vi "Accel_Test.vi"() -> ()   [LabVIEW 2015]
uses:
  <vilib>/myRIO/Instrument Drivers/Onboard Devices/Accelerometer/typedefs/Accelerometer Reference.ctl
  <vilib>/myRIO/Common/Instrument Driver Framework/Utilities/typedefs/myRIO Generic Hardware Reference.ctl
  <vilib>/myRIO/Common/Instrument Driver Framework/Utilities/typedefs/Hardware Version Enum.ctl
  <vilib>/myRIO/Common/Instrument Driver Framework/Utilities/typedefs/myRIO v1.0 Reference.ctl
  <vilib>/myRIO/Common/Instrument Driver Framework/Utilities/typedefs/Generic FPGA Reference.ctl
  <vilib>/myRIO/Common/Instrument Driver Framework/myRIO v1.0/Accelerometer/typedefs/Accelerometer Channels List.ctl
  <vilib>/myRIO/Common/Instrument Driver Framework/myRIO v1.0/Accelerometer/typedefs/Accelerometer Channels Enum.ctl
  <vilib>/userdefined/High Color/nirio_resource_hc.ctl
  <vilib>/myRIO/Common/Instrument Driver Framework/Utilities/vis/Is FPGA Ref Available.vi
  <vilib>/myRIO/Common/Instrument Driver Framework/myRIO v1.0/Accelerometer/vis/myRIO v1.1 Open Accelerometer.vi
  <vilib>/myRIO/Instrument Drivers/Onboard Devices/Accelerometer/vis/Read.vi
  <vilib>/Analysis/8numeric.llb/1D Numeric Integration.vi
  <vilib>/myRIO/Common/Instrument Driver Framework/Utilities/vis/Validate Channels.vi
  <vilib>/myRIO/Common/Instrument Driver Framework/myRIO v1.0/Accelerometer/vis/myRIO v1.0 Reserve Accelerometer.vi
  <vilib>/myRIO/Common/Instrument Driver Framework/myRIO v1.0/Resource Manager/vis/myRIO v1.0 Reserve Channel List.vi
  <vilib>/myRIO/Common/Instrument Driver Framework/myRIO v1.0/Accelerometer/vis/myRIO v1.0 Build MUX Configuration Accelerometer.vi
  <vilib>/myRIO/Common/Instrument Driver Framework/myRIO v1.0/Resource Manager/vis/myRIO v1.0 Reserve Channel.vi
  <vilib>/myRIO/Common/Instrument Driver Framework/myRIO v1.0/Resource Manager/vis/myRIO v1.0 Unreserve Channel.vi
  <vilib>/myRIO/Common/Instrument Driver Framework/myRIO v1.0/Resource Manager/vis/myRIO v1.0 Build Mutex Name.vi
  <vilib>/Utility/VariantDataType/GetNumericInfo.vi
  <vilib>/Utility/error.llb/Error Cluster From Error Code.vi
  <vilib>/myRIO/Common/Instrument Driver Framework/myRIO v1.0/myRIO v1.1 Open.vi
  <vilib>/myRIO/Common/Instrument Driver Framework/myRIO v1.0/Accelerometer/vis/myRIO v1.0 Get Scaling Constant Accelerometer.vi
  <vilib>/myRIO/Common/Instrument Driver Framework/Utilities/vis/IO Manager.vi
  <vilib>/myRIO/Common/Instrument Driver Framework/Utilities/vis/Configuration Manager.vi
  <vilib>/myRIO/Common/Instrument Driver Framework/myRIO v1.0/myRIO v1.0 Close.vi
  <vilib>/myRIO/Common/Instrument Driver Framework/myRIO v1.0/Accelerometer/vis/myRIO v1.0 Read Accelerometer.vi
  <vilib>/myRIO/Express VI/Onboard Devices/Accelerometer/Accelerometer Express VI.xnode
  <vilib>/myRIO/Instrument Drivers/Onboard Devices/Accelerometer/vis/myRIO Accelerometer Open.xnode
  <vilib>/Analysis/NI_AALPro.lvlib
  <vilib>/myRIO/Instrument Drivers/Onboard Devices/Accelerometer/Accelerometer.lvlib
panel:
  out "Waveform Chart  Y  2":dbl(graph)
  out "X-Axis 3":dbl
  out "dX/dY  Chart 3":dbl(graph)
  out "x/y":dbl
  out "Waveform Chart  Y":dbl(graph)
  out "Y-Axis":dbl
  out "\"position\"":dbl(graph)
  out "Current V":dbl
  out "Current A":dbl
  out "dX":dbl(graph)
  out "dA":dbl(graph)
  out "Avg A":dbl(graph)
  in  "stop 2":bool
  out "X-Axis 2":dbl
  out "Waveform Chart 2":dbl(graph)
  out "Waveform Chart X":dbl(graph)
  out "X-Axis":dbl
  in  "stop":bool
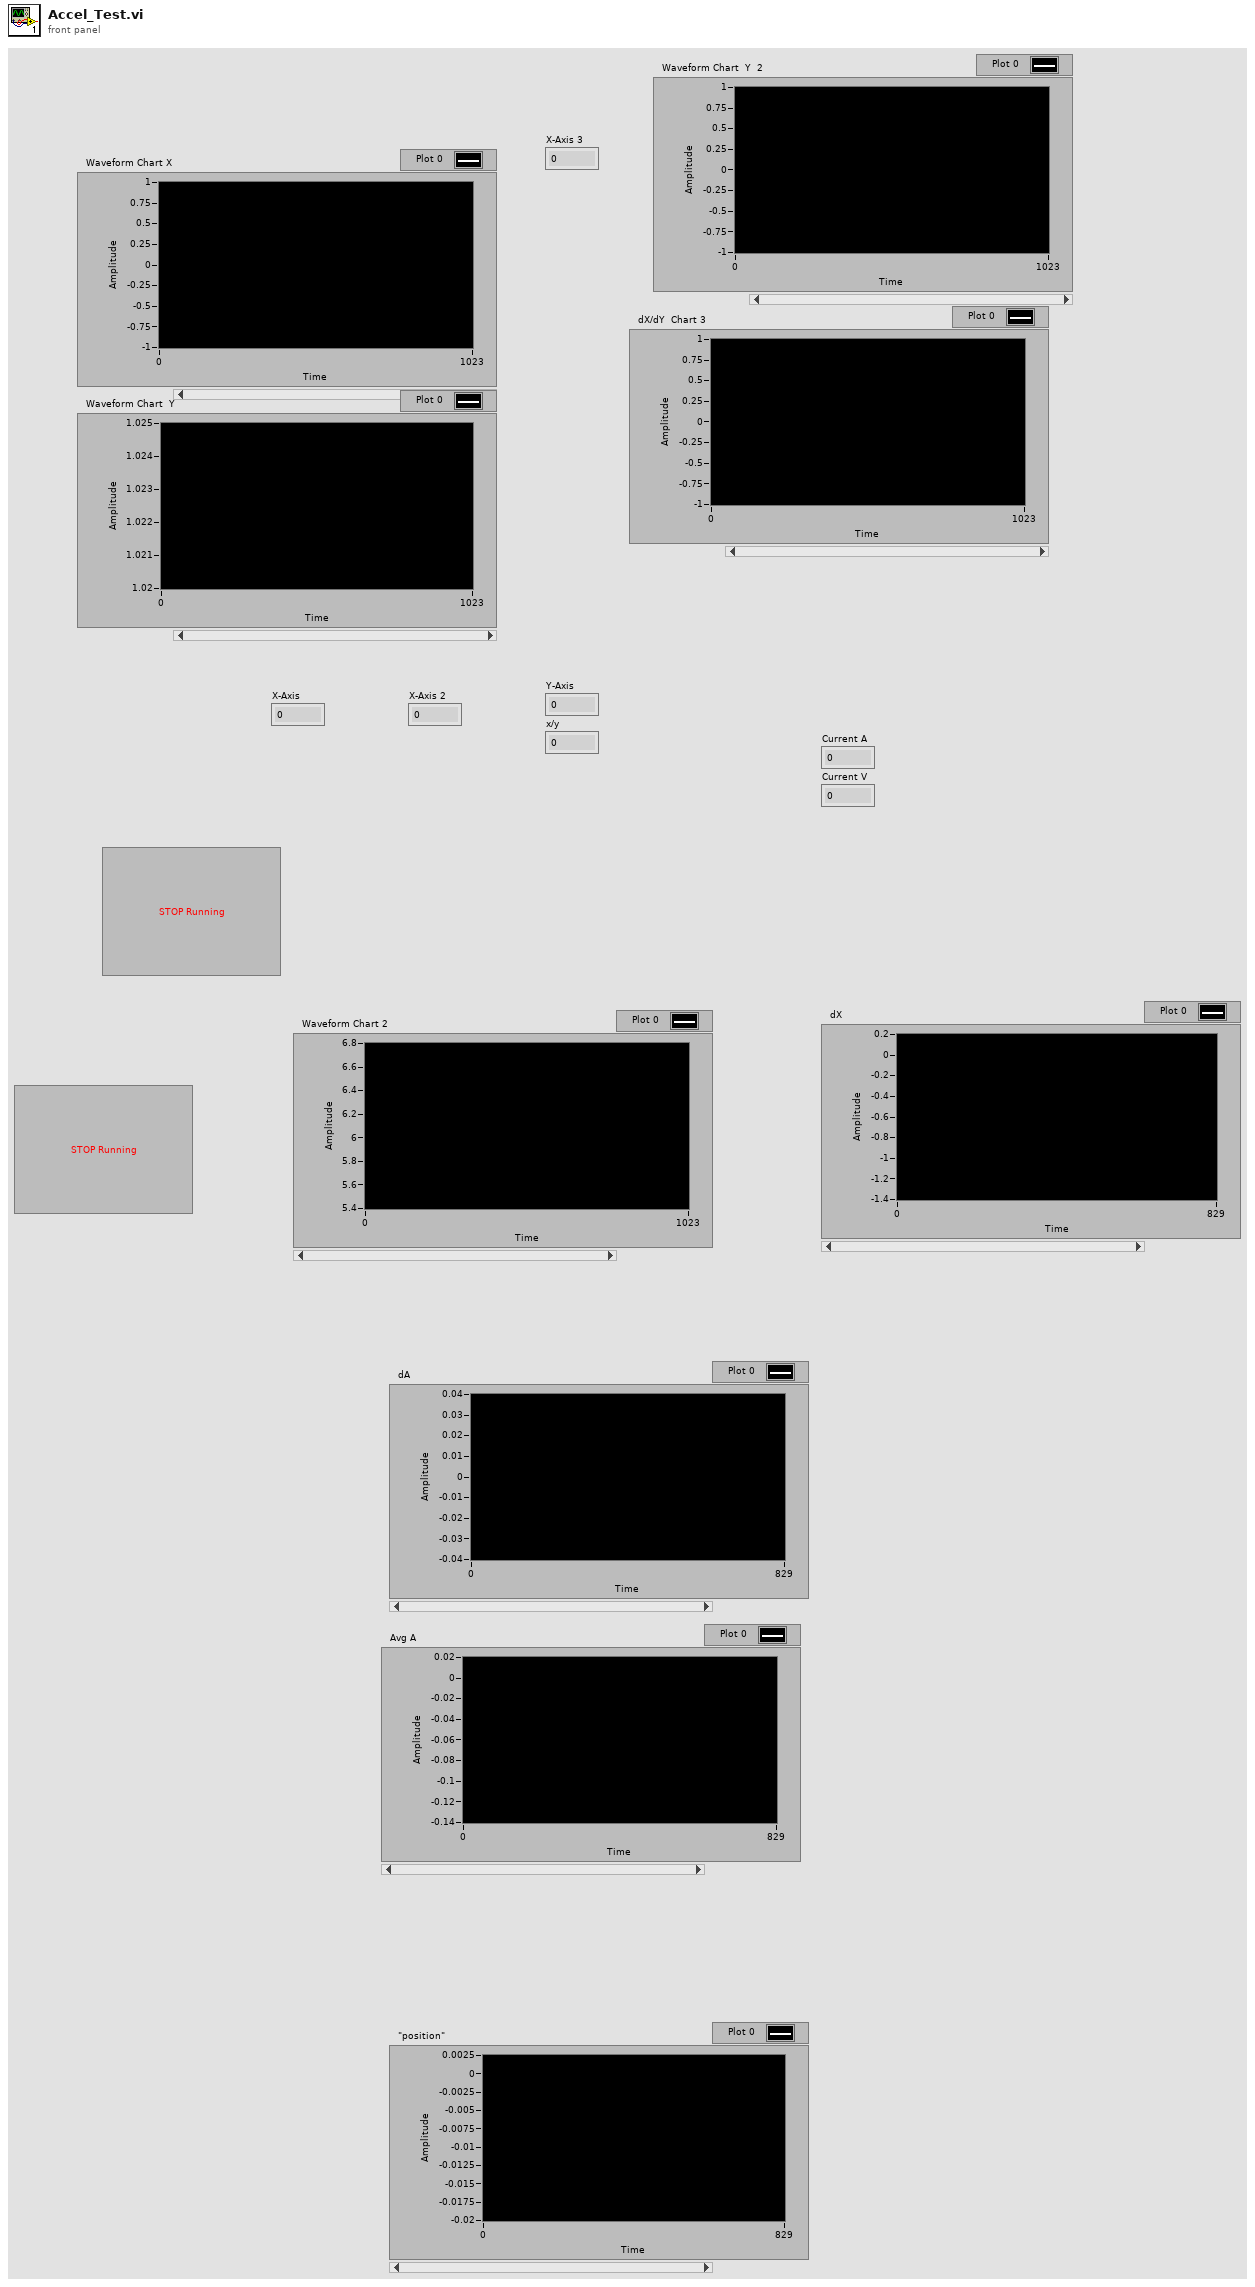
[diagram p1: front panel]
types:
  T1 = typedef "Accelerometer.lvlib/Accelerometer Reference.ctl" = cluster{"myRIO Reference":T2, "Accelerometer Channels List":T6, "LSB Weight":dbl}
  T2 = typedef "myRIO Generic Hardware Reference.ctl" = cluster{"myRIO Model":T3, "myRIO Hardware Reference":T4}
  T3 = typedef "Hardware Version Enum.ctl" = enum16{"Unknown", "myRIO-1900", "myRIO-1950", "roboRIO"}
  T4 = typedef "myRIO v1.0 Reference.ctl" = cluster{"Generic FPGA Reference":T5, "Allow multiple opens":bool}
  T5 = typedef "Generic FPGA Reference.ctl" = refnum<k20>
  T6 = typedef "Accelerometer Channels List.ctl" = T7[]
  T7 = typedef "Accelerometer Channels Enum.ctl" = enum16{"Not Connected", "X-Axis", "Y-Axis", "Z-Axis"}
  T8 = typedef "nirio_resource_hc.ctl" = tag
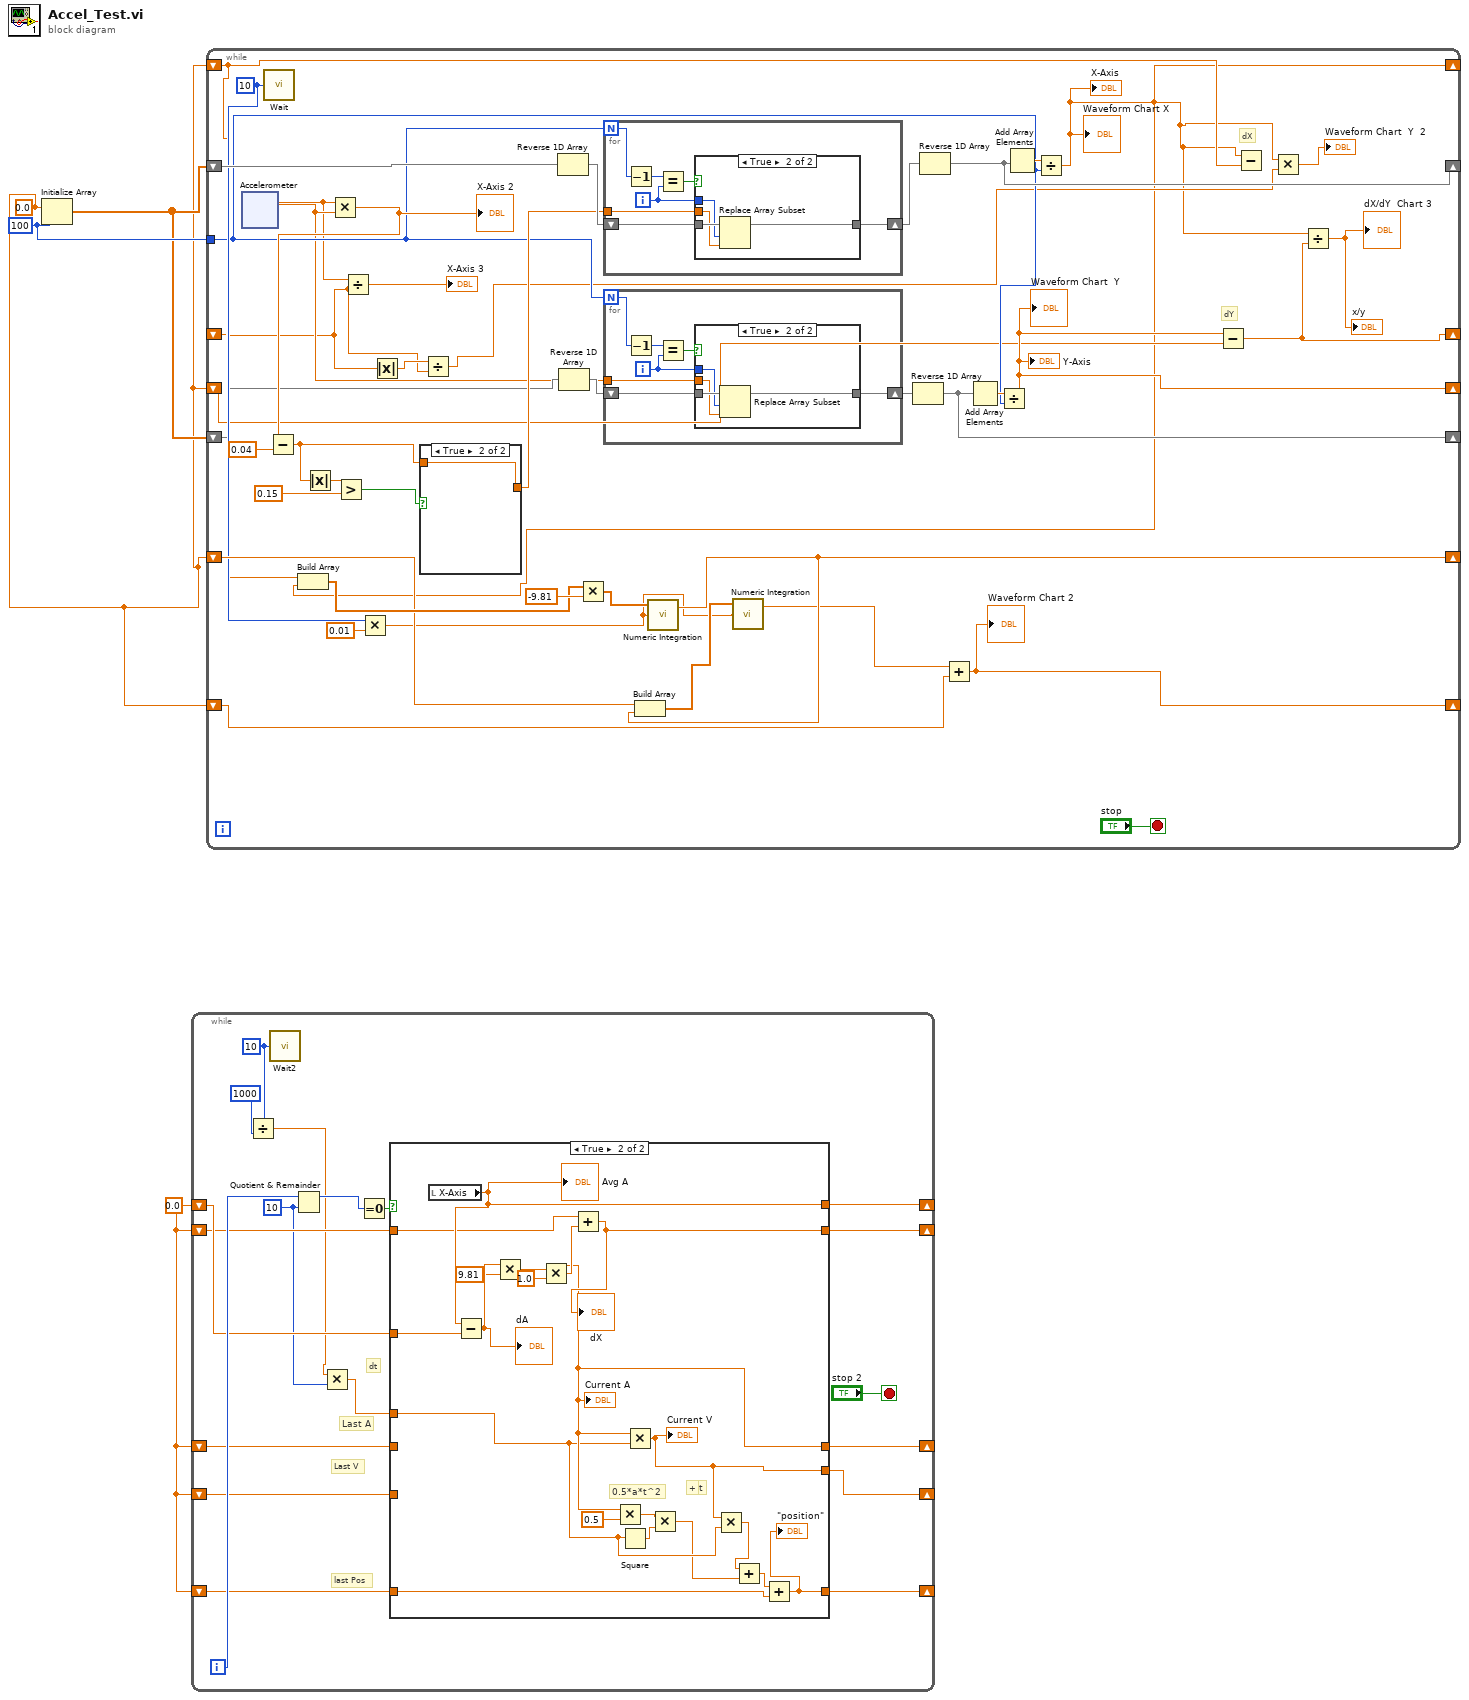
[diagram p0: block diagram]
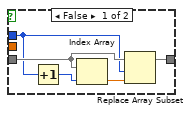
[diagram p3: hidden frame]
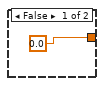
[diagram p4: hidden frame]
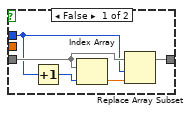
[diagram p5: hidden frame]
diagram:
  w3 = 0.0 ("X-Axis")
  w4 = 100 ("dimension size")
  w1 = 0.0 ("element")
  n1 = Initialize Array(w1, w4) -> (w2:dbl[])
  n2 = while {
    shift-right: [w19] -> _
    shift-left: w3 -> [w18]
    shift-right: [w17] -> _
    shift-left: w3 -> [w16]
    shift-right: [w15] -> _
    shift-left: w3 -> [w14]
    shift-right: [w7] -> _
    shift-left: w3 -> [w8]
    shift-right: [w6] -> _
    shift-left: w3 -> [w5]
    i -> [w20]
    stop <- "stop 2" stop-if-true
    w13 = u32 10 ("Count(mSec)")
    w10 = 10 ("y")
    # "last Pos"
    # "Last V"
    # "dt"
    # "Last A"
    n3 = Divide(x=w13, y=u32 1000) -> (x/y=w11:dbl)
    n4 = call "Wait2"("Count(mSec)"=w13) -> ()  [unwired: 1 out]
    n5 = Quotient & Remainder(x=w20, y=w10) -> (x-y*floor(x/y)=w21:i32)  [unwired: 1 out]
    n6 = Multiply(x=w11, y=w10) -> (x*y=w9:dbl)
    n7 = Equal To 0?(x=w21) -> (x = 0?=w22:bool)
    n8 = case shown="True" w22 {
      tunnel: [w28 w47] -> w19
      tunnel: w18 -> [w28 w46]
      tunnel: [w27 w40] -> w17
      tunnel: w16 -> [w27 w42]
      tunnel: [w26 w39] -> w15
      tunnel: w14 -> [w26 _]
      tunnel: w9 -> [_ w34]
      tunnel: w8 -> [w25 _]
      tunnel: [w25 w35] -> w7
      tunnel: [w24 w29] -> w6
      tunnel: w5 -> [w24 w30]
      frame False {
      }
      frame True {
        # "v*t"
        # "+"
        # "0.5*a*t^2"
        n9 = local read "X-Axis"() -> (w47:dbl)
        "Avg A" <- w47
        n10 = Subtract(x=w47, y=w46) -> (x-y=w45:dbl)
        "dA" <- w45
        n11 = Multiply(x=w45, y=9.81) -> (x*y=w39:dbl)
        "Current A" <- w39
        n12 = Multiply(x=w39, y=1.0) -> (x*y=w41:dbl)
        n13 = Add(x=w42, y=w41) -> (x+y=w40:dbl)
        "dX" <- w40
        n14 = Multiply(x=w39, y=0.5) -> (x*y=w37:dbl)
        n15 = Square(x=w34) -> (x^2=w36:dbl)
        n16 = Multiply(x=w39, y=w34) -> (x*y=w35:dbl)
        "Current V" <- w35
        n17 = Multiply(x=w37, y=w36) -> (x*y=w32:dbl)
        n18 = Multiply(x=w35, y=w34) -> (x*y=w33:dbl)
        n19 = Add(x=w33, y=w32) -> (x+y=w31:dbl)
        n20 = Add(x=w31, y=w30) -> (x+y=w29:dbl)
        "\"position\"" <- w29
      }
    }
  }
  n21 = while {
    shift-right: [w87] -> _
    shift-left: w2 -> [w85]
    tunnel: w4 -> [w64]
    shift-right: [w48] -> _
    shift-left: w1 -> [w59]
    shift-right: [w80] -> _
    shift-left: w1 -> [w81]
    shift-right: [w76] -> _
    shift-left: w1 -> [w78]
    shift-right: [w62] -> _
    shift-left: w2 -> [w63]
    shift-right: [w61] -> _
    shift-left: w1 -> [w60]
    shift-right: [w55] -> _
    shift-left: _ -> [w51]
    stop <- "stop" stop-if-true
    w74 = u32 10 ("Count(mSec)")
    # "dX"
    # "dY"
    n22 = xnode "Accelerometer"() -> ("X-Axis"=w54:dbl, "Y-Axis"=w56:dbl)  [unwired: 1 in, 1 out]
    n23 = call "Wait"("Count(mSec)"=w74) -> ()  [unwired: 1 out]
    n24 = Multiply(x=w54, y=w56) -> (x*y=w67:dbl)
    "X-Axis 2" <- w67
    n25 = Subtract(x=w67, y=0.04) -> (x-y=w68:dbl)
    n26 = Absolute Value(x=w68) -> (abs(x)=w72:dbl)
    n27 = Greater?(x=w72, y=0.15) -> (0:w71:bool)
    n28 = Divide(x=w54, y=w51) -> (x/y=→"X-Axis 3":dbl)
    n29 = Multiply(x=w74, y=0.01 ("element")) -> (x*y=w73:dbl)
    n30 = Absolute Value(x=w51) -> (abs(x)=w52:dbl)
    n31 = case shown="True" w71 {
      tunnel: [0.0 ("y") w109] -> w86
      tunnel: w68 -> [_ w109]
      frame False {
      }
      frame True {
      }
    }
    n32 = Divide(x=w52, y=w51) -> (x/y=w50:dbl)
    n33 = Reverse 1D Array(array=w85) -> (reversed array=w90:dbl[])
    n34 = Reverse 1D Array(array=w63) -> (reversed array=w57:dbl[])
    n35 = for {
      N: w64 -> [w115]
      shift-right: [w116] -> w89
      shift-left: w90 -> [w111]
      tunnel: w86 -> [w110]
      i -> [w112]
      n36 = Decrement(x=w115) -> (x-1=w113:i32)
      n37 = Equal?(x=w113, y=w112) -> (x = y?=w114:bool)
      n38 = case shown="True" w114 {
        tunnel: w112 -> [w118 w123]
        tunnel: w111 -> [w121 w124]
        tunnel: [w119 w125] -> w116
        tunnel: w110 -> [_ w122]
        frame False {
          n39 = Increment(x=w118) -> (x+1=w117:i32)
          n40 = Index Array(array=w121, index=w117) -> (element=w120:dbl)
          n41 = Replace Array Subset(array=w121, new element=w120, index=w118) -> (w119:dbl[])
        }
        frame True {
          n42 = Replace Array Subset(array=w124, new element=w122, index=w123) -> (w125:dbl[])
        }
      }
    }
    n43 = for {
      N: w64 -> [w97]
      shift-right: [w98] -> w66
      shift-left: w57 -> [w93]
      tunnel: w56 -> [w92]
      i -> [w94]
      n44 = Decrement(x=w97) -> (x-1=w95:i32)
      n45 = Equal?(x=w95, y=w94) -> (x = y?=w96:bool)
      n46 = case shown="True" w96 {
        tunnel: w94 -> [w100 w105]
        tunnel: w93 -> [w103 w106]
        tunnel: [w101 w107] -> w98
        tunnel: w92 -> [_ w104]
        frame False {
          n47 = Increment(x=w100) -> (x+1=w99:i32)
          n48 = Index Array(array=w103, index=w99) -> (element=w102:dbl)
          n49 = Replace Array Subset(array=w103, new element=w102, index=w100) -> (w101:dbl[])
        }
        frame True {
          n50 = Replace Array Subset(array=w106, new element=w104, index=w105) -> (w107:dbl[])
        }
      }
    }
    n51 = Reverse 1D Array(array=w66) -> (reversed array=w62:dbl[])
    n52 = Reverse 1D Array(array=w89) -> (reversed array=w87:dbl[])
    n53 = Add Array Elements(numeric array=w62) -> (sum=w65:dbl)
    n54 = Divide(x=w65, y=w64) -> (x/y=w61:dbl)
    "Y-Axis" <- w61
    "Waveform Chart  Y" <- w61
    n55 = Add Array Elements(numeric array=w87) -> (sum=w88:dbl)
    n56 = Divide(x=w88, y=w64) -> (x/y=w48:dbl)
    "X-Axis" <- w48
    "Waveform Chart X" <- w48
    n57 = Build Array(w59, w48) -> (w82:dbl[])
    n58 = Multiply(x=w82, y=-9.81 ("element")) -> (x*y=w83:dbl[])
    n59 = call-poly <vilib>:"Numeric Integration.vi"("dt"=w73, "Input Array"=w83) -> ("result"=w80:dbl)  [unwired: 1 in, 1 out]
    n60 = Build Array(w81, w80) -> (w79:dbl[])
    n61 = call-poly <vilib>:"Numeric Integration.vi"("dt"=w73, "Input Array"=w79) -> ("result"=w77:dbl)  [unwired: 1 in, 1 out]
    n62 = Add(x=w77, y=w78) -> (x+y=w76:dbl)
    "Waveform Chart 2" <- w76
    n63 = Subtract(x=w61, y=w60) -> (x-y=w55:dbl)
    n64 = Subtract(x=w48, y=w59) -> ()  [unwired: 1 out]
    n65 = Multiply(x=w48, y=w50) -> (x*y=→"Waveform Chart  Y  2":dbl)
    n66 = Divide(x=w48, y=w55) -> (x/y=→"x/y" →"dX/dY  Chart 3":dbl)
  }
